vi "Configure Instrument.vi"(0 "RFSG Session In":refnum<k15>, 5 "SG Configuration":T2={"Reference Clock Source"="OnboardClock", "Carrier Frequency (Hz)"=1000000000.0, "DUT Average Input Power (dBm)"=-20.0, "External Attenuation (dB)"=0.0, "SelectedPorts"=""} {"Carrier Frequency (Hz)" format="%#_6p"}, 7 "LO Configuration":T1={"LO Sharing Mode"=1, "LO Offset Mode"=1, "LO Offset (Hz)"=0.0} {"LO Offset Mode" items=["NoOffset", "Automatic", "User Defined"]; "LO Sharing Mode" items=["None", "Automatic", "Manual"]}, 11 "error in (no error)":errorcluster) -> (4 "RFSG Session Out":refnum<k15>, 15 "error out":errorcluster)   [LabVIEW 2016, in "SG.lvlib"]
uses:
  SG.lvlib
  Typedefs/Instrument Configuration.ctl
  <instrlib>/niRFSG/niRFSG.llb/niRFSG Ref Clock Sources.ctl
  Typedefs/LO Configruation.ctl
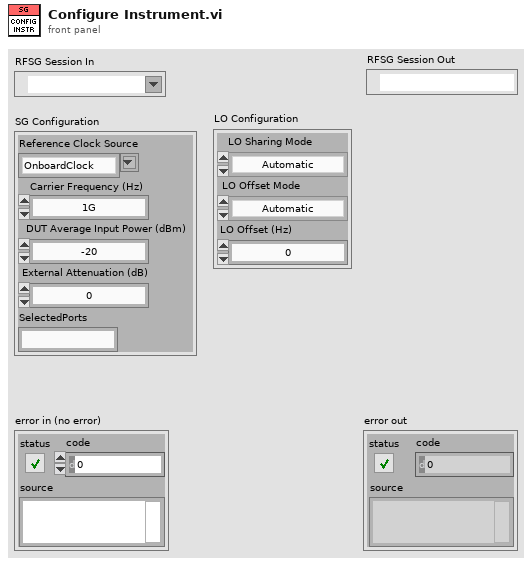
[diagram p1: front panel]
types:
  T1 = typedef "SG.lvlib/LO Configruation.ctl" = cluster{"LO Sharing Mode":i32, "LO Offset Mode":i32, "LO Offset (Hz)":dbl}
  T2 = typedef "SG.lvlib/Instrument Configuration.ctl" = cluster{"Reference Clock Source":T3, "Carrier Frequency (Hz)":dbl, "DUT Average Input Power (dBm)":dbl, "External Attenuation (dB)":dbl, "SelectedPorts":string}
  T3 = typedef "niRFSG Ref Clock Sources.ctl" = string
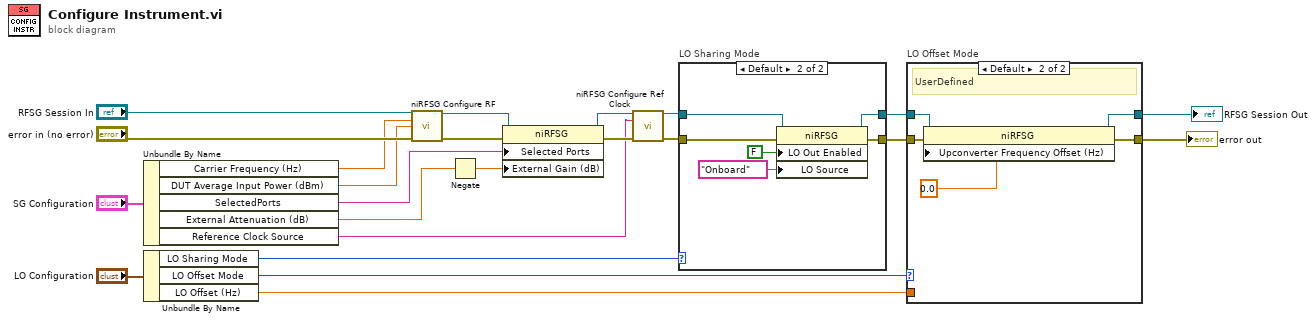
[diagram p0: block diagram]
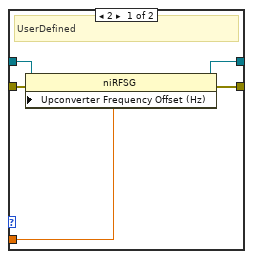
[diagram p2: hidden frame]
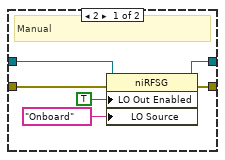
[diagram p3: hidden frame]
diagram:
  n1 = Unbundle By Name("SG Configuration") -> ("Carrier Frequency (Hz)"=w18:dbl, "DUT Average Input Power (dBm)"=w17:dbl, "SelectedPorts"=w9:string, "External Attenuation (dB)"=w14:dbl, "Reference Clock Source"=w11:T3)
  n2 = Unbundle By Name("LO Configuration") -> ("LO Sharing Mode"=w7:i32, "LO Offset Mode"=w5:i32, "LO Offset (Hz)"=w4:dbl)
  n3 = call <instrlib>:"niRFSG Configure RF.vi"("instrument handle"="RFSG Session In", "frequency (Hz)"=w18, "power level (dBm)"=w17, "error in"="error in (no error)") -> ("instrument handle out"=w16:refnum<k15>, "error out"=w22:errorcluster)  [unwired: 10 in]
  n4 = Negate(x=w14) -> (-x=w10:dbl)
  n5 = property class="niRFSG"(reference=w16, error in=w22, "Selected Ports"=w9, "External Gain (dB)"=w10) -> (reference out=w15:refnum<k15>, error out=w21:errorcluster)
  n6 = call <instrlib>:"niRFSG Configure Ref Clock.vi"("instrument handle"=w15, "ref clock source"=w11, "error in"=w21) -> ("instrument handle out"=w13:refnum<k15>, "error out"=w12:errorcluster)  [unwired: 11 in]
  n7 = case "LO Sharing Mode" shown="Default" w7 {
    tunnel: w12 -> [w29 w35]
    tunnel: w13 -> [w27 w33]
    tunnel: [w28 w34] -> w3
    tunnel: [w26 w32] -> w6
    frame 2 {
      # "Manual"
      n8 = property class="niRFSG"(reference=w27, error in=w29, "LO Out Enabled"=TRUE ("RF:LO Out Enabled"), "LO Source"="Onboard" ("Device Specific:Vector Signal Transceiver:Signal Path:LO Source")) -> (reference out=w26:refnum<k15>, error out=w28:errorcluster)
    }
    frame Default {
      n9 = property class="niRFSG"(reference=w33, error in=w35, "LO Out Enabled"=FALSE ("RF:LO Out Enabled"), "LO Source"="Onboard" ("Device Specific:Vector Signal Transceiver:Signal Path:LO Source")) -> (reference out=w32:refnum<k15>, error out=w34:errorcluster)
    }
  }
  n10 = case "LO Offset Mode" shown="Default" w5 {
    tunnel: w3 -> [w40 w45]
    tunnel: w6 -> [w38 w43]
    tunnel: [w39 w44] -> w2
    tunnel: [w37 w42] -> w1
    tunnel: w4 -> [w36 _]
    frame 2 {
      # "UserDefined"
      n11 = property class="niRFSG"(reference=w38, error in=w40, "Upconverter Frequency Offset (Hz)"=w36) -> (reference out=w37:refnum<k15>, error out=w39:errorcluster)
    }
    frame Default {
      # "UserDefined"
      n12 = property class="niRFSG"(reference=w43, error in=w45, "Upconverter Frequency Offset (Hz)"=0.0 ("Device Specific:Vector Signal Transceiver:Upconverter:Frequency Offset (Hz)")) -> (reference out=w42:refnum<k15>, error out=w44:errorcluster)
    }
  }
  "error out" <- w2
  "RFSG Session Out" <- w1
